vi "Power Multiplicator.vi"(10 "Iteration i":dbl) -> (2 "Coefficient":dbl)   [LabVIEW 2012]
doc: "This VI calculates the power coeeficient to be exactly:\n\n i coeff\n 0 100% of power\n 1 75% of power\n 2 50% of power\n 3 25 % of power\n 4 0 % of power"
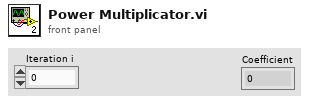
[diagram p1: front panel]
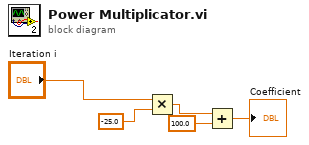
[diagram p0: block diagram]
diagram:
  n1 = Multiply(x="Iteration i", y=-25.0) -> (x*y=w3:dbl)
  n2 = Add(x=w3, y=100.0) -> (x+y=→"Coefficient":dbl)
